vi "Read Type.vi"(8 "Error In":errorcluster, 11 "Text In":refnum<class "Text.lvclass">) -> (0 "Error Out":errorcluster, 2 "Type":T1=enum."Unknown", 3 "Text Out":refnum<class "Text.lvclass">)   [LabVIEW 2018, in "Toolkit.lvlib" / "Nodes.lvlib" / "Text.lvclass"]
doc: "Gets the Node type. LabVIEW 2009 does not have the Get LV Class Name function, so this is a workaround to determine the Node class/type during run-time."
uses:
  Text.lvclass
  Type Definitions/Types.ctl
  Nodes.lvlib
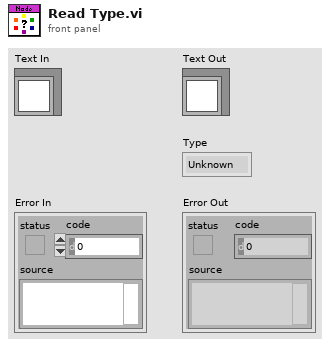
[diagram p1: front panel]
types:
  T1 = typedef "Toolkit.lvlib/Nodes.lvlib/Types.ctl" = enum16{"Comment", "Delimiter", "Partial", "Root", "Section", "Text", "Unknown", "Variable"}
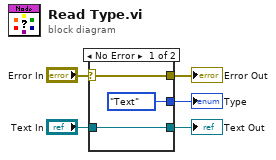
[diagram p0: block diagram]
diagram:
  n1 = case shown="No Error" "Error In" {
    selector: "Error In" -> [w8 w10]
    tunnel: [w8 w10] -> w4
    tunnel: [w7 w9] -> w3
    tunnel: "Text In" -> [w7 w9]
    tunnel: [Types."Text" ("Type") _] -> w1
    frame No Error {
    }
    frame Error {
    }
  }
  "Error Out" <- w4
  "Text Out" <- w3
  "Type" <- w1
